vi "Init.vi"(5 "host":string="localhost", 7 "lib":string="TrendAnaliserEng", 9 "update timeout":dbl, 11 "error in (no error)":errorcluster) -> (4 "SVW":refnum<class "SharedVariableWrapper.lvclass">, 15 "error out":errorcluster)   [LabVIEW 2019, in "SharedVariableWrapper.lvclass"]
uses:
  SharedVariableWrapper.lvclass
  shared variable info.ctl
  Config.ctl
  SharedVariableWrapper.lvclass/SharedVariableWrapper.ctl
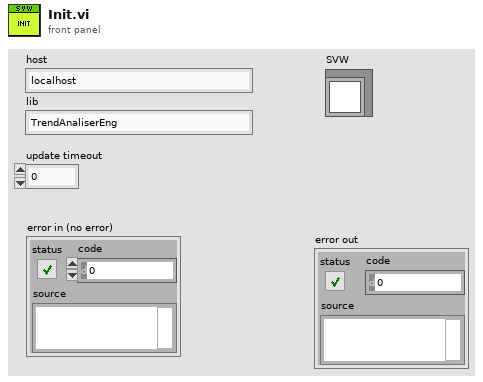
[diagram p1: front panel]
types:
  T1 = typedef "SharedVariableWrapper.lvclass/Config.ctl" = cluster{"connection str":string, "timeout":dbl, "ip":string}
  T2 = typedef "SharedVariableWrapper.lvclass/shared variable info.ctl" = cluster{"shared variable":refnum<k21>, "connected":bool, "Value":variant, "UpdateTime":timestamp}
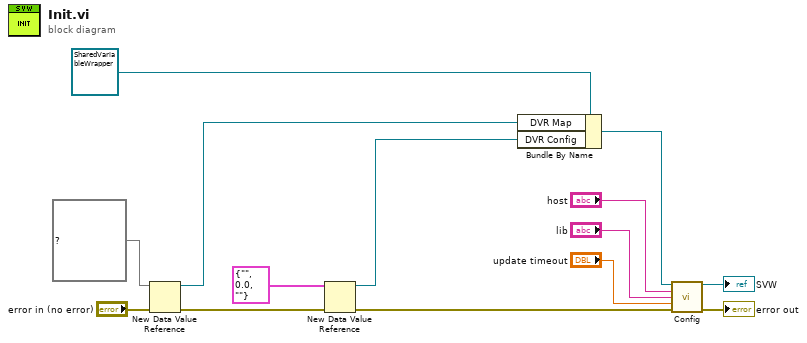
[diagram p0: block diagram]
diagram:
  n1 = New Data Value Reference(data value=map{string, T2} {} ("map"), error in="error in (no error)") -> (data value reference=w12:refnum<data-value>, error out=w6:errorcluster)
  n2 = New Data Value Reference(data value=T1 {"connection str"="", "timeout"=0.0, "ip"=""} ("Config"), error in=w6) -> (data value reference=w2:refnum<data-value>, error out=w5:errorcluster)
  n3 = Bundle By Name(cluster=refnum<class "SharedVariableWrapper.lvclass"> refnum ("SharedVariableWrapper in"), "DVR Map"=w12, "DVR Config"=w2) -> (w8:refnum<class "SharedVariableWrapper.lvclass">)
  n4 = call "Config.vi"("SharedVariableWrapper in"=w8, "host"="host", "lib"="lib", "update timeout"="update timeout", "error in"=w5) -> ("SharedVariableWrapper"=→"SVW":refnum<class "SharedVariableWrapper.lvclass">, "error out"=→"error out":errorcluster)  [unwired: 9 in]
